vi "testUDPReciever - Copy.vi"() -> ()   [LabVIEW 2012]
panel:
  out "in 11":bool
  out "in 10":bool
  out "in 9":bool
  out "in 8":bool
  out "in 7":bool
  out "in 6":bool
  out "in 5":bool
  out "in 4":bool
  out "in 3":bool
  out "in 2":bool
  out "in 1":bool
  out "in 0":bool
  out "NumBins":u32
  out "Cnts/Bin":u32
  out "Prof/Hist":u32
  out "Sync":u32
  out "Channel":u32
  out "rTime":u32
  out "frameCntr":u32
  out "built packet array":string[](array[string])
  out "channel":u32
  out "built header":bool[][](array[boolean])
  out "Found Header":bool
  out "Raw Data Out":string
  out "error post-check":errorcluster
  out "End Reciever Error":errorcluster
  in  "stop reciever":bool
  out "port":u16
  out "error out post-read":errorcluster
  out "error out pre-read":errorcluster
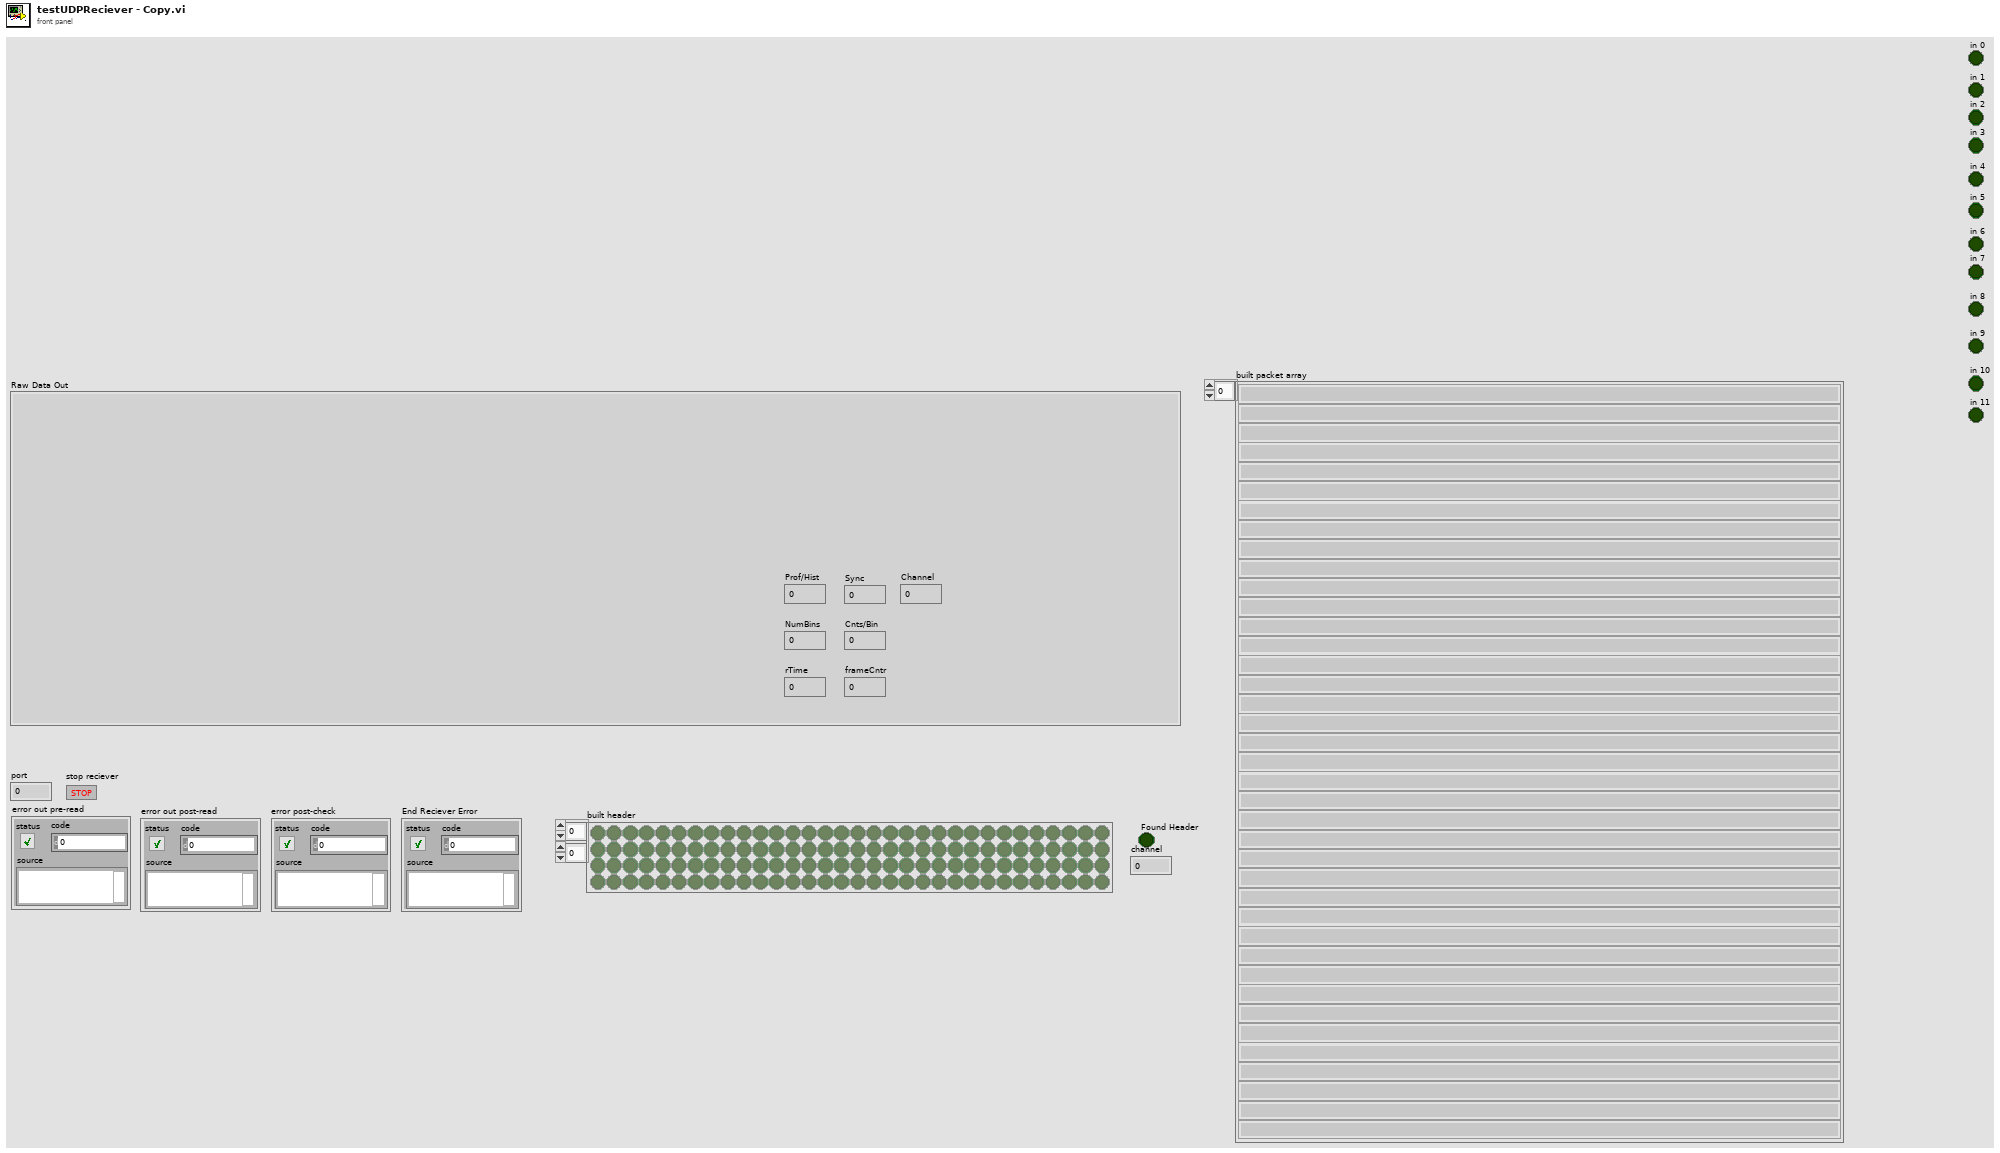
[diagram p1: front panel]
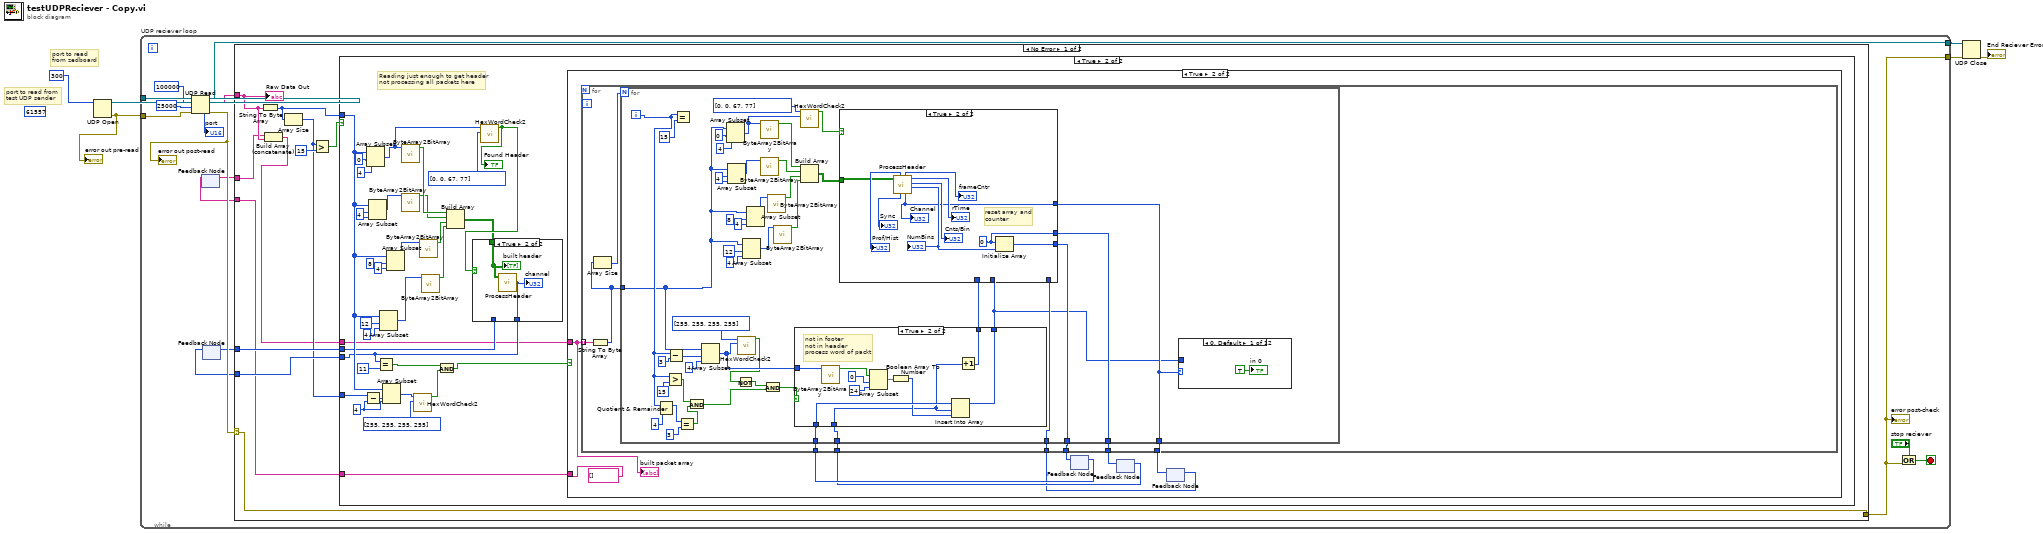
[diagram p0: block diagram]
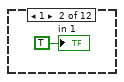
[diagram p4: hidden frame]
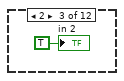
[diagram p5: hidden frame]
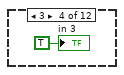
[diagram p6: hidden frame]
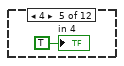
[diagram p7: hidden frame]
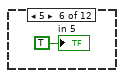
[diagram p8: hidden frame]
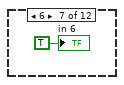
[diagram p9: hidden frame]
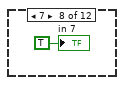
[diagram p10: hidden frame]
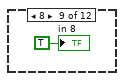
[diagram p11: hidden frame]
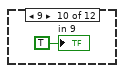
[diagram p12: hidden frame]
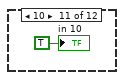
[diagram p13: hidden frame]
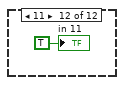
[diagram p14: hidden frame]
diagram:
  (unwired) u16 61557 ("port")
  # "port to read \nfrom zedboard"
  # "port to read from \ntest UDP sender"
  n1 = UDP Open(11:u16 300 ("port")) -> (port=w5:refnum<k16>, 0:w2:errorcluster)  [unwired: 4 in, 1 out]
  "error out pre-read" <- w2
  n2 = while "UDP reciever loop" {
    tunnel: [w21] -> w6
    tunnel: w5 -> [w20]
    tunnel: [w12] -> w4
    tunnel: w2 -> [w17]
    stop <- w19 stop-if-true
    n3 = UDP Read(connection ID=w20, max size (548)=100000, timeout ms (25000)=25000, 8:w17) -> (data out=w14:string, error out=w16:errorcluster, 3:w21:refnum<k16>, 4:→"port":u16)  [unwired: 1 out]
    "error out post-read" <- w16
    n4 = feedback #1() -> (w9:string[])  [unwired: 1 in]
    n5 = feedback #2() -> (w7:u32)  [unwired: 1 in]
    n6 = case shown="No Error" w16 {
      selector: w16 -> [w32 w171]
      tunnel: w14 -> [w31 _]
      tunnel: [w32 w171] -> w12
      tunnel: [w22 w170] -> w10
      tunnel: w9 -> [w30 w170]
      tunnel: [w27 w169] -> w8
      tunnel: w7 -> [w26 w169]
      frame No Error {
        n7 = String To Byte Array(string=w31) -> (unsigned byte array=w23:u8[])
        n8 = Build Array (concatenate)(w30, w31) -> (w24:string[])
        n9 = Array Size(array=w23) -> (size(s)=w25:i32)
        n10 = Greater?(x=w25, y=15) -> (0:w29:bool)
        n11 = case shown="True" w29 {
          tunnel: w23 -> [_ w45]
          tunnel: [w34 w38] -> w27
          tunnel: w26 -> [w34 w39]
          tunnel: w25 -> [_ w42]
          tunnel: w24 -> [w33 w36]
          tunnel: [w33 w35] -> w22
          frame False {
          }
          frame True {
            w44 = 4 ("length")
            w61 = 4 ("length")
            # "Reading just enough to get header\nnot processing all packets here"
            n12 = Subtract(x=w42, y=w44) -> (x-y=w43:i32)
            n13 = Array Subset(array=w45, index=0, length=4) -> (w50:u8[])
            n14 = Array Subset(array=w45, index=w61, length=w61) -> (w66:u8[])
            n15 = Array Subset(array=w45, index=12, length=4) -> (w48:u8[])
            n16 = Array Subset(array=w45, index=w43, length=w44) -> (w37:u8[])
            n17 = Array Subset(array=w45, index=8, length=4) -> (w65:u8[])
            n18 = call "ByteArray2BitArray.vi"("array"=w50) -> ("Array"=w56:bool[])  [unwired: 10 in]
            n19 = call "ByteArray2BitArray.vi"("array"=w66) -> ("Array"=w55:bool[])  [unwired: 10 in]
            n20 = call "HexWordCheck2.vi"("array"=u8[] [255, 255, 255, 255], "Input Array"=w37) -> ("Boolean"=w46:bool)  [unwired: 9 in]
            n21 = call "ByteArray2BitArray.vi"("array"=w65) -> ("Array"=w53:bool[])  [unwired: 10 in]
            n22 = call "ByteArray2BitArray.vi"("array"=w48) -> ("Array"=w54:bool[])  [unwired: 10 in]
            n23 = Build Array(w56, w55, w53, w54) -> (w51:bool[][])
            n24 = call "HexWordCheck2.vi"("array"=u8[] [0, 0, 67, 77], "Input Array"=w50) -> ("Boolean"=w52:bool)  [unwired: 9 in]
            "Found Header" <- w52
            n25 = case shown="True" w52 {
              tunnel: w51 -> [_ w168]
              tunnel: [w166 w167] -> w38
              tunnel: w39 -> [w166 _]
              frame False {
              }
              frame True {
                n26 = call "ProcessHeader.vi"("Array"=w168) -> ("Numeric 4"=w167:u32)  [unwired: 4 in, 6 out]
                "channel" <- w167
                "built header" <- w168
              }
            }
            n27 = Equal?(x=w38, y=u32 11) -> (x = y?=w41:bool)
            n28 = And(x=w41, y=w46) -> (x .and. y?=w47:bool)
            n29 = case shown="True" w47 {
              tunnel: w36 -> [w67 w68]
              tunnel: [w67 string[] []] -> w35
              frame False {
              }
              frame True {
                n30 = feedback #3() -> (w74:u32[])  [unwired: 1 in]
                n31 = feedback #4() -> (w72:u32)  [unwired: 1 in]
                n32 = feedback #5() -> (w70:u32)  [unwired: 1 in]
                n33 = for {
                  tunnel: w68 -> [w84] mode=indexing
                  tunnel: [w79] -> w75
                  tunnel: w74 -> [w78]
                  tunnel: [w81] -> w73
                  tunnel: w72 -> [w82]
                  tunnel: [w80] -> w71
                  tunnel: w70 -> [w83]
                  n34 = String To Byte Array(string=w84) -> (unsigned byte array=w77:u8[])
                  n35 = Array Size(array=w77) -> (size(s)=w76:i32)
                  n36 = for {
                    N: w76 -> [_]
                    tunnel: w77 -> [w93]
                    tunnel: w83 -> [w92]
                    tunnel: [w89] -> w80
                    tunnel: w82 -> [w91]
                    tunnel: [w90] -> w81
                    tunnel: [w88] -> w79
                    tunnel: w78 -> [w87]
                    i -> [w94]
                    w108 = 4 ("length")
                    n37 = Quotient & Remainder(x=w94, y=4) -> (x-y*floor(x/y)=w124:i32)  [unwired: 1 out]
                    n38 = Greater?(x=w94, y=15 ("x")) -> (0:w126:bool)
                    n39 = Subtract(x=w94, y=3) -> (x-y=w120:i32)
                    n40 = Equal?(x=w94, y=15) -> ()  [unwired: 1 out]
                    n41 = Equal?(x=w124, y=3 ("x")) -> (x = y?=w125:bool)
                    n42 = And(x=w126, y=w125) -> (x .and. y?=w117:bool)
                    n43 = Array Subset(array=w93, index=w120, length=4) -> (w115:u8[])
                    n44 = Array Subset(array=w93, index=0, length=4) -> (w98:u8[])
                    n45 = Array Subset(array=w93, index=w108, length=w108) -> (w112:u8[])
                    n46 = call "HexWordCheck2.vi"("array"=w115, "Input Array"=u8[] [255, 255, 255, 255] ("array")) -> ("Boolean"=w113:bool)  [unwired: 9 in]
                    n47 = Not(x=w113) -> (.not. x?=w114:bool)
                    n48 = Array Subset(array=w93, index=12, length=4) -> (w99:u8[])
                    n49 = Array Subset(array=w93, index=8, length=4) -> (w111:u8[])
                    n50 = call "ByteArray2BitArray.vi"("array"=w112) -> ("Array"=w102:bool[])  [unwired: 10 in]
                    n51 = call "ByteArray2BitArray.vi"("array"=w98) -> ("Array"=w103:bool[])  [unwired: 10 in]
                    n52 = And(x=w114, y=w117) -> (x .and. y?=w116:bool)
                    n53 = call "ByteArray2BitArray.vi"("array"=w111) -> ("Array"=w100:bool[])  [unwired: 10 in]
                    n54 = call "ByteArray2BitArray.vi"("array"=w99) -> ("Array"=w101:bool[])  [unwired: 10 in]
                    n55 = case shown="True" w116 {
                      tunnel: w87 -> [w142 w152]
                      tunnel: w91 -> [w141 w144]
                      tunnel: w115 -> [_ w146]
                      tunnel: [w142 w145] -> w85
                      tunnel: [w141 w143] -> w86
                      frame False {
                      }
                      frame True {
                        # "not in footer \nnot in header\nprocess word of packt"
                        n56 = call "ByteArray2BitArray.vi"("array"=w146) -> ("Array"=w147:bool[])  [unwired: 10 in]
                        n57 = Array Subset(array=w147, index=0, length=24) -> (w149:bool[])
                        n58 = Boolean Array To Number(Boolean array=w149) -> (number=w148:u32)
                        n59 = Insert Into Array(array=w152, index=w144, new element=w148) -> (w145:u32[])
                        n60 = Increment(x=w144) -> (x+1=w143:u32)
                      }
                    }
                    n61 = call "HexWordCheck2.vi"("array"=w98, "Input Array"=u8[] [0, 0, 67, 77] ("array")) -> ("Boolean"=w96:bool)  [unwired: 9 in]
                    n62 = Build Array(w103, w102, w100, w101) -> (w95:bool[][])
                    n63 = case shown="True" w96 {
                      tunnel: w95 -> [_ w159]
                      tunnel: [w155 w158] -> w88
                      tunnel: [w154 w157] -> w90
                      tunnel: w85 -> [w155 _]
                      tunnel: w86 -> [w154 _]
                      tunnel: [w153 w156] -> w89
                      tunnel: w92 -> [w153 _]
                      frame False {
                        # "not in header, so process start of packet"
                      }
                      frame True {
                        w157 = u32 0 ("element")
                        # "reset array and \ncounter"
                        n64 = call "ProcessHeader.vi"("Array"=w159) -> ("Numeric"=w160:u32, "Numeric 7"=→"Cnts/Bin":u32, "Numeric 3"=→"rTime":u32, "Numeric 4"=w156:u32, "Numeric 2"=→"frameCntr":u32, "Numeric 5"=→"Sync":u32, "Numeric 6"=→"Prof/Hist":u32)  [unwired: 4 in]
                        "NumBins" <- w160
                        "Channel" <- w156
                        n65 = Initialize Array(w157, w160) -> (w158:u32[])
                      }
                    }
                    n66 = case shown="0, Default" w89 {
                      tunnel: w85 -> [_ _ _ _ _ _ _ _ _ _ _ _]
                      frame 0, Default {
                        "in 0" <- TRUE ("in 11")
                      }
                      frame 1 {
                        "in 1" <- TRUE ("in 11")
                      }
                      frame 2 {
                        "in 2" <- TRUE ("in 11")
                      }
                      frame 3 {
                        "in 3" <- TRUE ("in 11")
                      }
                      frame 4 {
                        "in 4" <- TRUE ("in 11")
                      }
                      frame 5 {
                        "in 5" <- TRUE ("in 11")
                      }
                      frame 6 {
                        "in 6" <- TRUE ("in 11")
                      }
                      frame 7 {
                        "in 7" <- TRUE ("in 11")
                      }
                      frame 8 {
                        "in 8" <- TRUE ("in 11")
                      }
                      frame 9 {
                        "in 9" <- TRUE ("in 11")
                      }
                      frame 10 {
                        "in 10" <- TRUE ("in 11")
                      }
                      frame 11 {
                        "in 11" <- TRUE ("in 11")
                      }
                    }
                  }
                }
                n67 = feedback-in #3(w75) -> ()
                n68 = feedback-in #4(w73) -> ()
                n69 = feedback-in #5(w71) -> ()
                "built packet array" <- w68
              }
            }
          }
        }
        "Raw Data Out" <- w31
      }
      frame Error {
      }
    }
    "error post-check" <- w12
    n70 = feedback-in #1(w10) -> ()
    n71 = feedback-in #2(w8) -> ()
    n72 = Or(x="stop reciever", y=w12) -> (x .or. y?=w19:bool)
  }
  n73 = UDP Close(connection ID=w6, 8:w4) -> (error out=→"End Reciever Error":errorcluster)  [unwired: 1 out]
